vi "fgv_8-bit export AVI mode.vi"(8 "error in (no error)":errorcluster, 9 "Function":enum16{"Intialize", "Write", "Read", "Clear"}(ring), 11 "AVI mode":T1) -> (0 "error out":errorcluster, 3 "AVI mode":T1)   [LabVIEW 2013]
uses:
  Typedefs/AVI implementation enum.ctl
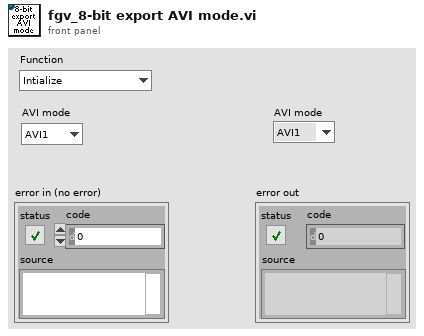
[diagram p1: front panel]
types:
  T1 = typedef "AVI implementation enum.ctl" = enum16{"AVI1", "AVI2"}
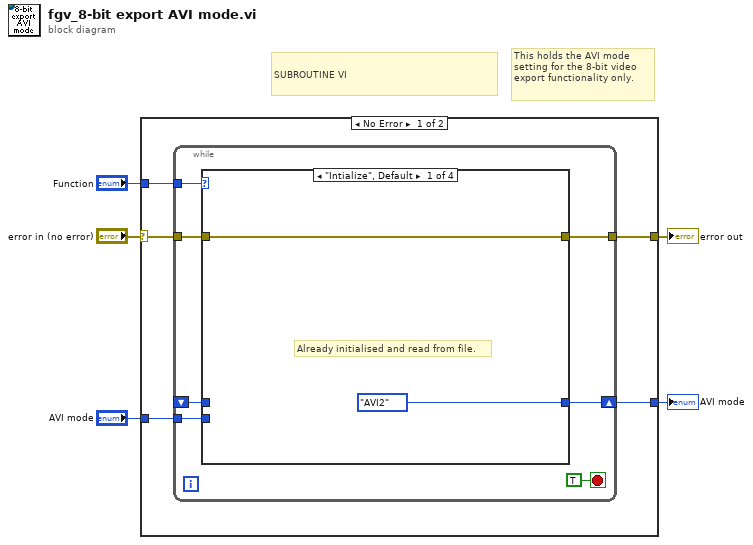
[diagram p0: block diagram]
diagram:
  # "This holds the AVI mode setting for the 8-bit video export functionality only."
  # "SUBROUTINE VI"
  n1 = case shown="No Error" "error in (no error)" {
    selector: "error in (no error)" -> [w8 w26]
    tunnel: [w9 w26] -> w4
    tunnel: "Function" -> [w10 _]
    tunnel: "AVI mode" -> [w7 w25]
    tunnel: [w6 w25] -> w1
    frame No Error {
      n2 = while {
        tunnel: w10 -> [w16]
        tunnel: [w14] -> w9
        tunnel: w8 -> [w15]
        tunnel: w7 -> [w13]
        shift-right: [w12] -> w6
        shift-left: _ -> [w11]
        stop <- TRUE stop-if-true
        n3 = case shown="\"Intialize\", Default" w16 {
          tunnel: [w19 w21 w23 w24] -> w14
          tunnel: w15 -> [w19 w21 w23 w24]
          tunnel: w13 -> [_ w20 _ _]
          tunnel: [AVI_implementation_enum."AVI2" ("AVI mode") w20 w22 _] -> w12
          tunnel: w11 -> [_ _ w22 _]
          frame "Intialize", Default {
            # "Already initialised and read from file."
          }
          frame "Write" {
          }
          frame "Read" {
          }
          frame "Clear" {
          }
        }
      }
    }
    frame Error {
    }
  }
  "error out" <- w4
  "AVI mode" <- w1
